vi "UpLo Convertor.vi"(11 "triangle matrix type":T2=3 items=["Lower Triangular"=2, "Upper Triangular"=3]) -> (3 "uplo":T1=121 items=["CblasUpper"=121, "CblasLower"=122])   [LabVIEW 2020, in "NI_AALBLAS.lvlib"]
uses:
  <vilib>/Analysis/NI_AALBLAS.lvlib
  <vilib>/Analysis/BLAS.llb/LV_UpLo.ctl
  <vilib>/Analysis/BLAS.llb/UpLo.ctl
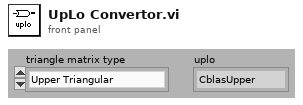
[diagram p1: front panel]
types:
  T1 = typedef "NI_AALBLAS.lvlib/UpLo.ctl" = i32
  T2 = typedef "NI_AALBLAS.lvlib/LV_UpLo.ctl" = i32
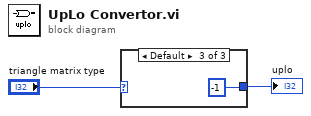
[diagram p0: block diagram]
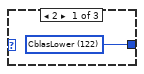
[diagram p2: hidden frame]
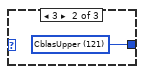
[diagram p3: hidden frame]
diagram:
  n1 = case shown="Default" "triangle matrix type" {
    tunnel: [w3 w4 -1] -> w2
    frame 2 {
      w3 = T1 122 items=["CblasUpper"=121, "CblasLower"=122] ("uplo 2")
    }
    frame 3 {
      w4 = T1 121 items=["CblasUpper"=121, "CblasLower"=122] ("uplo 2")
    }
    frame Default {
    }
  }
  "uplo" <- w2
